vi "pessimize_objective_fun_ucno.vi"(3 "output control":T1, 4 "data":T2, 5 "X":dbl[](array[numeric])) -> (0 "error out":errorcluster, 1 "gradient":dbl[](array[numeric]), 2 "f(X)":dbl)   [LabVIEW 2013]
doc: "This template is the starting point for creating an objectivel function to be passed to the Unconstrained Optimization.vi."
uses:
  <vilib>/gmath/NumericalOptimization/objective function data.ctl
  <vilib>/gmath/NI_Gmath.lvlib
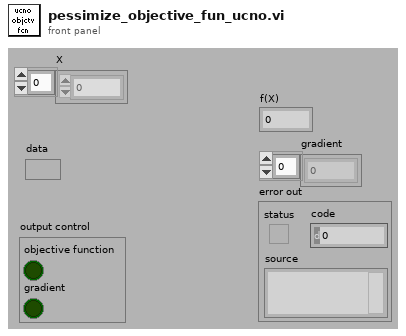
[diagram p1: front panel]
types:
  T1 = cluster{"objective function":bool, "gradient":bool}
  T2 = typedef "NI_Gmath.lvlib/objective function data.ctl" = variant
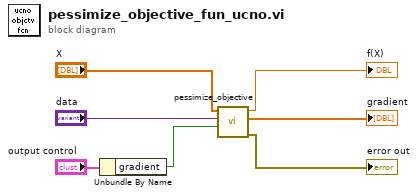
[diagram p0: block diagram]
diagram:
  n1 = Unbundle By Name("output control") -> ("gradient"=w2:bool)
  n2 = call "pessimize_objective.vi"("Find gradient"=w2, "data"="data", "X"="X") -> ("error out"=→"error out":errorcluster, "Gradient"=→"gradient":dbl[], "f(X)"=→"f(X)":dbl)  [unwired: 6 in]
